vi "PutNil.vi"(8 "error in (no error)":errorcluster, 11 "MsgPackSerializer in":refnum<class "MsgPackSerializer.lvclass">) -> (0 "error out":errorcluster, 3 "MsgPackSerializer out":refnum<class "MsgPackSerializer.lvclass">)   [LabVIEW 2015, in "MsgPackSerializer.lvclass"]
uses:
  MsgPackSerializer.lvclass
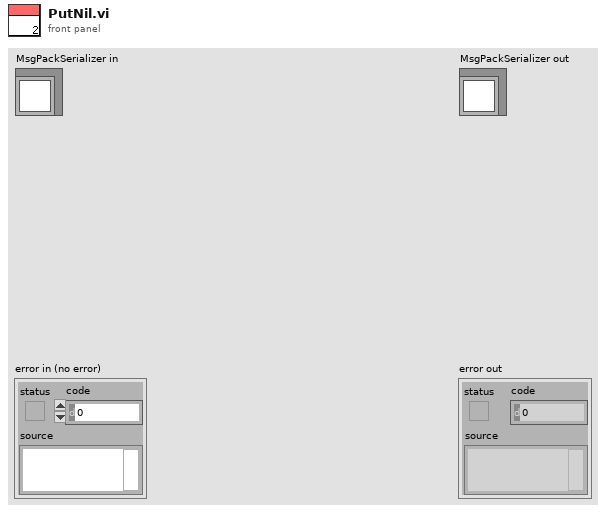
[diagram p1: front panel]
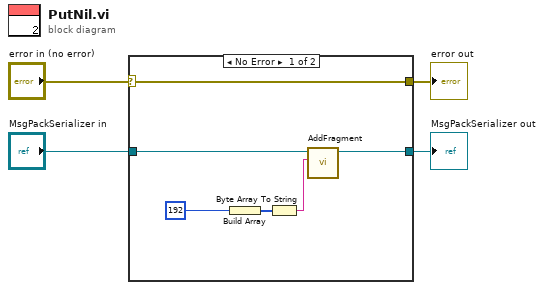
[diagram p0: block diagram]
diagram:
  n1 = case shown="No Error" "error in (no error)" {
    selector: "error in (no error)" -> [w10 w12]
    tunnel: [w10 w12] -> w3
    tunnel: [w8 w11] -> w1
    tunnel: "MsgPackSerializer in" -> [w9 w11]
    frame No Error {
      n2 = Build Array(u8 192 ("Number")) -> (w6:u8[])
      n3 = Byte Array To String(unsigned byte array=w6) -> (string=w5:string)
      n4 = call "AddFragment.vi"("Fragment"=w5, "MsgPackSerializer in"=w9) -> ("MsgPackSerializer out"=w8:refnum<class "MsgPackSerializer.lvclass">)  [unwired: 8 in, 1 out]
    }
    frame Error {
    }
  }
  "error out" <- w3
  "MsgPackSerializer out" <- w1
